vi "DefineAction.vi"(8 "ErrorIn":errorcluster, 9 "Measurement":refnum<class "IAction.lvclass">, 10 "Name":string, 11 "TopModuleIn":refnum<class "TopModule.lvclass">) -> (0 "ErrorOut":errorcluster, 3 "TopModuleOut":refnum<class "TopModule.lvclass">)   [LabVIEW 2019, in "TopModule.lvclass"]
uses:
  TopModule.lvclass
  IAction/IAction.lvclass
  TopModule.lvclass/TopModule.ctl
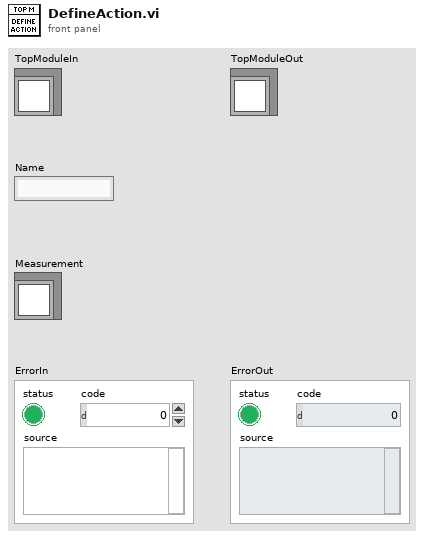
[diagram p1: front panel]
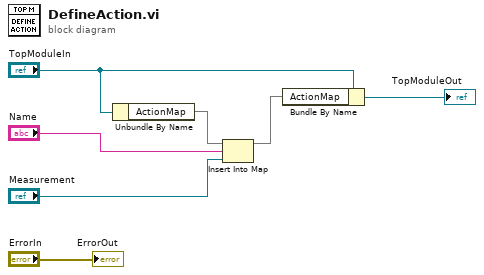
[diagram p0: block diagram]
diagram:
  n1 = Unbundle By Name("TopModuleIn") -> ("ActionMap"=w5:map{string, refnum<class "IAction.lvclass">})
  n2 = Insert Into Map(map in=w5, key="Name", value="Measurement") -> (map out=w6:map{string, refnum<class "IAction.lvclass">})  [unwired: 2 out]
  n3 = Bundle By Name(cluster="TopModuleIn", "ActionMap"=w6) -> (→"TopModuleOut":refnum<class "TopModule.lvclass">)
  "ErrorOut" <- "ErrorIn"
